vi "Obtain update state data event.vi"(8 "error in (no error)":errorcluster) -> (0 "error out":errorcluster, 3 "Update state data":refnum<user-event>)   [LabVIEW 2018, in "Fiber Auto Collimation References.lvclass"]
doc: "This VI gets the reference to an event that should be fired from the Model loop every time the state data changes, and sent to the View loops on all running panels to change any readouts that derive from some part of the state data."
uses:
  Fiber Auto Collimation References.lvclass
  State data/Fiber Auto Collimation state data.lvclass
  C:/Program Files (x86)/National Instruments/LabVIEW 2018/user.lib/nLight Tidbits/Cross-library references/Cross-library key/Cross-library key.lvclass
  2c7179bb-cec4-496a-af02-303d080efcd1.vi
  654a22ce-1768-4d71-8b6d-67a80da22744.vi
  2c7179bb-cec4-496a-af02-303d080efcd1.vi/94c69346-51e4-4bdb-9046-53562b4fe964.vi
  <userlib>/nLight Tidbits/Cross-library references/Cross-library key/Obtain cross library semaphore and acquire.vi
  2c7179bb-cec4-496a-af02-303d080efcd1.vi/e3b70d98-1d71-4502-a942-9fe56d633078.vi
  654a22ce-1768-4d71-8b6d-67a80da22744.vi/f1259e42-7d77-4267-a9f6-72d752ddc996.vi
  654a22ce-1768-4d71-8b6d-67a80da22744.vi/904a9240-cb72-4973-b8c7-bb05da90f8f3.vi
  <userlib>/nLight Error Handling/Trash error.vi
  <vilib>/Utility/error.llb/Clear Errors.vi
  <vilib>/Utility/semaphor.llb/Obtain Semaphore Reference.vi
  <vilib>/Utility/semaphor.llb/Acquire Semaphore.vi
  <userlib>/nLight Error Handling/Log any errors.vi
  <userlib>/nLight Tidbits/Cross-library references/Cross-library key/Obtain class key.vi
  <vilib>/Utility/semaphor.llb/Release Semaphore.vi
  <vilib>/Utility/semaphor.llb/Release Semaphore Reference.vi
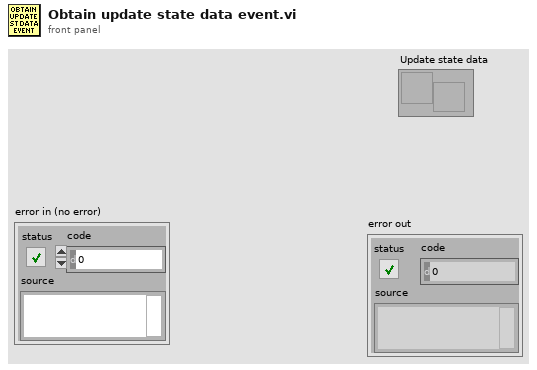
[diagram p1: front panel]
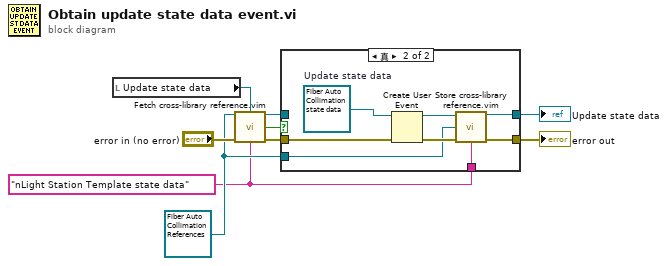
[diagram p0: block diagram]
diagram:
  w1 = "nLight Station Template state data"
  w3 = refnum<class "Fiber Auto Collimation References.lvclass"> refnum ("nLight Station Template References.lvclass")
  n1 = local read "Update state data"() -> (w5:refnum<user-event>)
  n2 = call "Fetch cross-library reference.vim"("Cross-library key"=w3, "Reference type to fetch"=w5, "error in (no error)"="error in (no error)", "Specific ref type name [String/Enum]"=w1) -> ("Stored value (if present)"=w4:refnum<user-event>, "Nothing to fetch OR bad reference"=w2:bool, "error out"=w6:errorcluster)  [unwired: 9 in]
  n3 = case shown="真" w2 {
    tunnel: w6 -> [w10 w19]
    tunnel: [w10 w13] -> w8
    tunnel: [w11 w14] -> w9
    tunnel: w4 -> [w11 _]
    tunnel: w3 -> [_ w16]
    tunnel: w1 -> [_ w12]
    frame False {
    }
    frame True {
      w18 = refnum<class "Fiber Auto Collimation state data.lvclass"> refnum  # Update state data
      n4 = Create User Event(user event datatype=w18, error in=w19) -> (user event=w15:refnum<user-event>, error out=w17:errorcluster)
      n5 = call "Store cross-library reference.vim"("Reference to store"=w15, "Cross-library key"=w16, "error in (no error)"=w17, "Specific ref type name [String/Enum]"=w12) -> ("Copy of stored reference"=w14:refnum<user-event>, "error out"=w13:errorcluster)  [unwired: 8 in, 2 out]
    }
  }
  "error out" <- w8
  "Update state data" <- w9
